vi "Construct Run Tests Step.vi"(5 "Run Tests Step in":refnum<class "Run Tests Step.lvclass">, 8 "error in (no error)":errorcluster, 11 "Path":path) -> (0 "error out":errorcluster, 3 "Run Tests Step":refnum<class "Run Tests Step.lvclass">)   [LabVIEW 2019, in "Caraya Library.lvlib" / "Run Tests Step.lvclass"]
uses:
  Run Tests Step.lvclass
  Run Tests Step.lvclass/Run Tests Step.ctl
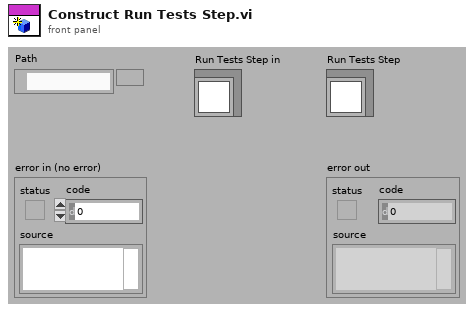
[diagram p1: front panel]
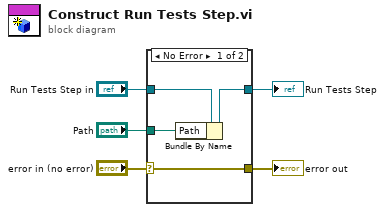
[diagram p0: block diagram]
diagram:
  n1 = case shown="No Error" "error in (no error)" {
    selector: "error in (no error)" -> [w9 w11]
    tunnel: [w9 w11] -> w4
    tunnel: [w7 w10] -> w2
    tunnel: "Run Tests Step in" -> [w8 w10]
    tunnel: "Path" -> [w6 _]
    frame No Error {
      n2 = Bundle By Name(cluster=w8, "Path"=w6) -> (w7:refnum<class "Run Tests Step.lvclass">)
    }
    frame Error {
    }
  }
  "error out" <- w4
  "Run Tests Step" <- w2
